vi "strict.getXMLTestSuite.vi"(9 "indent level":i32, 10 "testsuite":T1={"name"="", "errors"=0, "skipped"=0, "tests"=0, "failures"=0, "time"=-1.0, "timestamp"=timestamp(0 s since 1904-01-01), "properties"=[], "Call Chain"=[]}) -> (1 "testsuite (end)":string="</testsuite>", 2 "testsuite (start)":string[](array[string]))   [LabVIEW 2013, in "strict-JUnit.lvclass"]
uses:
  strict-JUnit.lvclass
  <vilib>/addons/_JKI Toolkits/Caraya/classes/Test Report.JUnit/testsuite -- cluster.ctl
  <vilib>/addons/_JKI Toolkits/Caraya/classes/Test Report.JUnit/property -- cluster.ctl
  <vilib>/addons/_JKI Toolkits/Caraya/classes/Test Report/Test Report.lvclass
  <vilib>/addons/_JKI Toolkits/Caraya/classes/Test Report.JUnit/Test Report.JUnit.lvclass
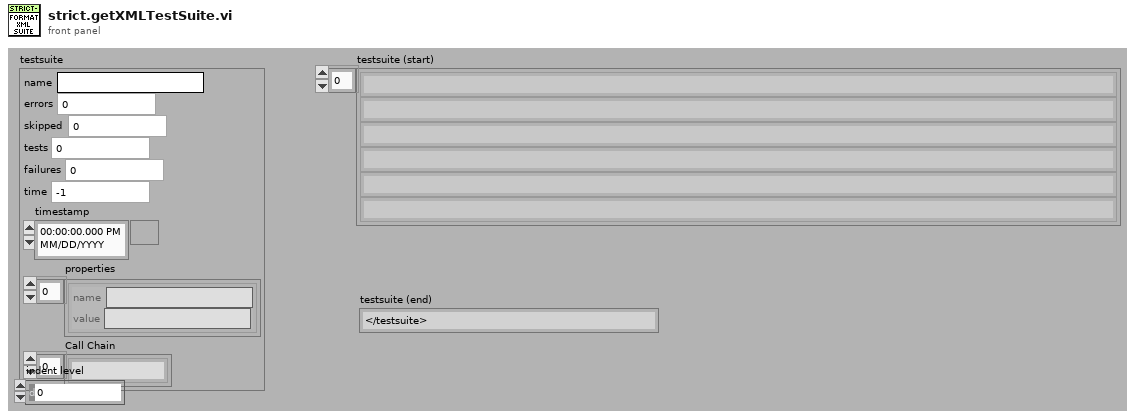
[diagram p1: front panel]
types:
  T1 = typedef "Caraya.lvlib/Test Report.JUnit.lvclass/testsuite -- cluster.ctl" = cluster{"name":string, "errors":u32, "skipped":u32, "tests":u32, "failures":u32, "time":dbl, "timestamp":timestamp, "properties":T2[], "Call Chain":string[]}
  T2 = typedef "Caraya.lvlib/Test Report.JUnit.lvclass/property -- cluster.ctl" = cluster{"name":string, "value":string}
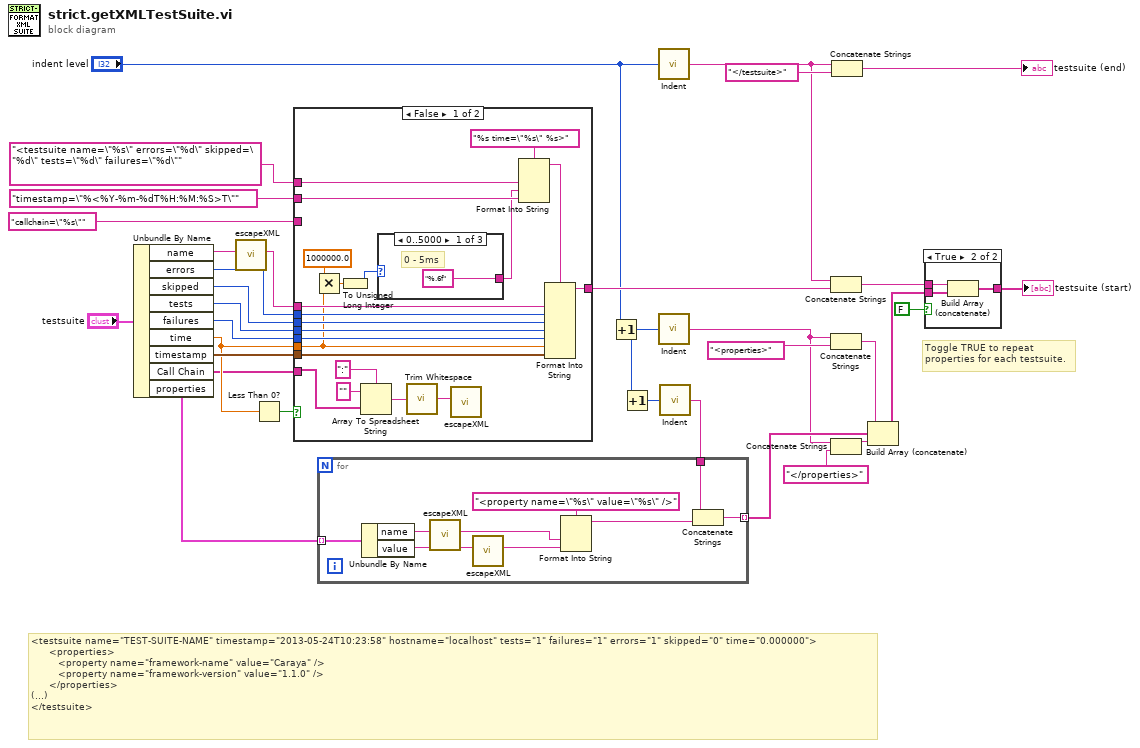
[diagram p0: block diagram]
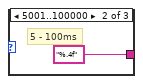
[diagram p2: hidden frame]
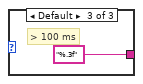
[diagram p3: hidden frame]
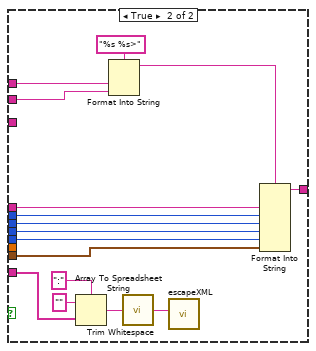
[diagram p4: hidden frame]
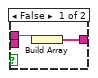
[diagram p5: hidden frame]
diagram:
  # "<testsuite name=\"TEST-SUITE-NAME\" timestamp=\"2013-05-24T10:23:58\" hostname=\"localhost\" tests=\"1\" failures=\"1\" errors=\"1\" skipped=\"0\" time=\"0.000000\">\n      <properties>\n         <property name=\"framework-name\" value=\"Caraya\" />\n         <property name=\"framework-version\" value=\"1.1.0\" />\n      </properties>\n(...)\n</testsuite>"
  # "Toggle TRUE to repeat\nproperties for each testsuite."
  n1 = Unbundle By Name("testsuite") -> ("name"=w4:string, "errors"=w32:u32, "skipped"=w30:u32, "tests"=w29:u32, "failures"=w28:u32, "time"=w8:dbl, "timestamp"=w27:timestamp, "Call Chain"=w2:string[], "properties"=w26:T2[])
  n2 = call <vilib>:"escapeXML.vi"("Input String"=w4) -> ("XML-escaped String"=w3:string)  [unwired: 10 in]
  n3 = Less Than 0?(x=w8) -> (x < 0?=w7:bool)
  n4 = case shown="False" w7 {
    tunnel: w32 -> [w54 w73]
    tunnel: w3 -> [w53 w72]
    tunnel: w30 -> [w52 w71]
    tunnel: w29 -> [w51 w70]
    tunnel: w28 -> [w50 w69]
    tunnel: w27 -> [w49 w68]
    tunnel: [w48 w67] -> w23
    tunnel: w8 -> [w43 _]
    tunnel: "<testsuite name=\"%s\" errors=\"%d\" skipped=\"%d\" tests=\"%d\" failures=\"%d\"" -> [w47 w66]
    tunnel: "timestamp=\"%<%Y-%m-%dT%H:%M:%S>T\"" -> [w46 w65]
    tunnel: w2 -> [w38 w59]
    tunnel: "callchain=\"%s\"" -> [_ _]
    frame False {
      n5 = Multiply(x=1000000.0 ("y"), y=w43) -> (x*y=w41:dbl)
      n6 = To Unsigned Long Integer(number=w41) -> (unsigned 32bit integer=w40:u32)
      n7 = Array To Spreadsheet String(delimiter (Tab)=":" ("format string"), array=w38, 3:"" ("format string")) -> (spreadsheet string=w35:string)
      n8 = case shown="0..5000" w40 {
        tunnel: ["%.6f" "%.4f" "%.3f"] -> w39
        frame 0..5000 {
          # "0 - 5ms"
        }
        frame 5001..100000 {
          # "5 - 100ms"
        }
        frame Default {
          # "> 100 ms"
        }
      }
      n9 = call <vilib>:"Trim Whitespace.vi"("string"=w35) -> ("trimmed string"=w34:string)  [unwired: 1 in]
      n10 = call <vilib>:"escapeXML.vi"("Input String"=w34) -> ()  [unwired: 10 in, 1 out]
      n11 = Format Into String(format string="%s time=\"%s\" %s>", w47, w39, w46) -> (resulting string=w44:string)  [unwired: 2 in, 1 out]
      n12 = Format Into String(format string=w44, w53, w54, w52, w51, w50, w43, w49) -> (resulting string=w48:string)  [unwired: 2 in, 1 out]
    }
    frame True {
      n13 = Array To Spreadsheet String(delimiter (Tab)=":" ("format string"), array=w59, 3:"" ("format string")) -> (spreadsheet string=w60:string)
      n14 = Format Into String(format string="%s %s>", w66, w65) -> (resulting string=w64:string)  [unwired: 2 in, 1 out]
      n15 = call <vilib>:"Trim Whitespace.vi"("string"=w60) -> ("trimmed string"=w58:string)  [unwired: 1 in]
      n16 = call <vilib>:"escapeXML.vi"("Input String"=w58) -> ()  [unwired: 10 in, 1 out]
      n17 = Format Into String(format string=w64, w72, w73, w71, w70, w69, w68) -> (resulting string=w67:string)  [unwired: 2 in, 1 out]
    }
  }
  n18 = Increment(x="indent level") -> (x+1=w12:i32)
  n19 = Increment(x=w12) -> (x+1=w10:i32)
  n20 = call <vilib>:"Indent.vi"("Numeric"="indent level") -> ("string"=w13:string)
  n21 = call <vilib>:"Indent.vi"("Numeric"=w12) -> ("string"=w11:string)
  n22 = call <vilib>:"Indent.vi"("Numeric"=w10) -> ("string"=w9:string)
  n23 = for {
    tunnel: w26 -> [w82] mode=indexing
    tunnel: [w79] -> w24 mode=indexing
    tunnel: w9 -> [w78]
    n24 = Unbundle By Name(w82) -> ("name"=w77:string, "value"=w75:string)
    n25 = call <vilib>:"escapeXML.vi"("Input String"=w77) -> ("XML-escaped String"=w76:string)  [unwired: 10 in]
    n26 = call <vilib>:"escapeXML.vi"("Input String"=w75) -> ("XML-escaped String"=w74:string)  [unwired: 10 in]
    n27 = Format Into String(format string="<property name=\"%s\" value=\"%s\" />", w76, w74) -> (resulting string=w80:string)  [unwired: 2 in, 1 out]
    n28 = Concatenate Strings(w78, w80) -> (w79:string)
  }
  n29 = Concatenate Strings(w13, w23) -> (w22:string)
  n30 = Concatenate Strings(w11, "<properties>") -> (w20:string)
  n31 = Concatenate Strings(w11, "</properties>") -> (w19:string)
  n32 = Concatenate Strings(w13, "</testsuite>" ("testsuite (end)")) -> (→"testsuite (end)":string)
  n33 = Build Array (concatenate)(w20, w24, w19) -> (w25:string[])
  n34 = case shown="True" FALSE {
    tunnel: [w83 w87] -> w33
    tunnel: w25 -> [_ w86]
    tunnel: w22 -> [w84 w85]
    frame False {
      n35 = Build Array(w84) -> (w83:string[])
    }
    frame True {
      n36 = Build Array (concatenate)(w85, w86) -> (w87:string[])
    }
  }
  "testsuite (start)" <- w33
